vi "Alarm Clock.vi"() -> ()   [LabVIEW 2015]
uses:
  Control 1.ctl
panel:
  in  "Alarm Time":timestamp
  out "Alarm set for":timestamp
  out "Current Time":timestamp
  in  "Turn OFF":bool
  in  "OFF":bool
  in  "Set Alarm":bool
  in  "Snooze":bool
  out "Alarm":bool
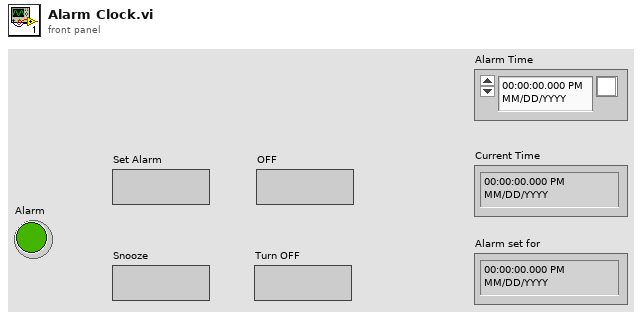
[diagram p1: front panel]
types:
  T1 = typedef "Control 1.ctl" = enum16{"Evaluate", "Set Alarm", "Alarm on", "Alarm off", "Snooze"}
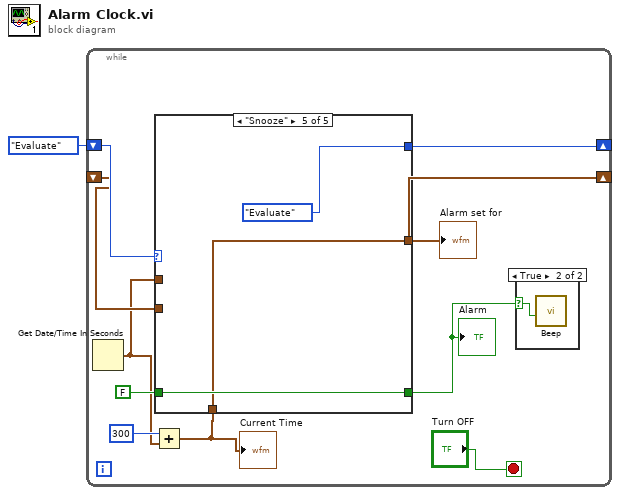
[diagram p0: block diagram]
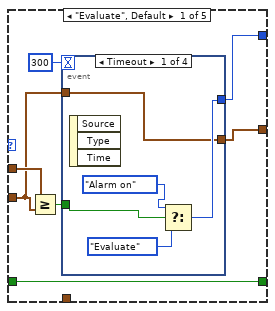
[diagram p3: hidden frame]
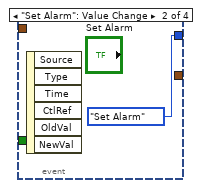
[diagram p4: hidden frame]
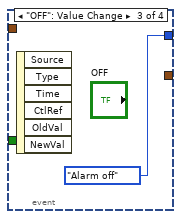
[diagram p5: hidden frame]
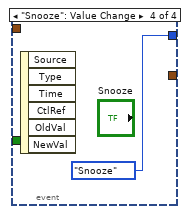
[diagram p6: hidden frame]
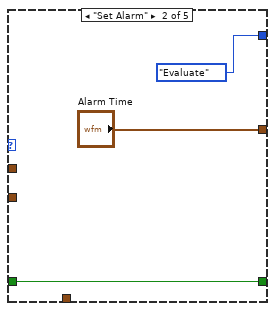
[diagram p7: hidden frame]
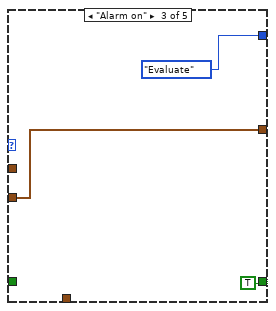
[diagram p8: hidden frame]
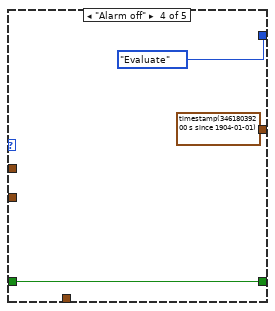
[diagram p9: hidden frame]
diagram:
  n1 = while {
    shift-right: [w9] -> _
    shift-left: Control_1."Evaluate" -> [w11]
    shift-right: [w10] -> _
    shift-left: _ -> [w8]
    stop <- "Turn OFF" stop-if-true
    n2 = Get Date/Time In Seconds() -> (seconds since 1Jan1904=w4:timestamp)
    n3 = Add(x=300, y=w4) -> (x+y=w3:timestamp)
    "Current Time" <- w3
    n4 = case shown="\"Snooze\"" w11 {
      tunnel: [w13 "Alarm Time" w32 timestamp(34618039200 s since 1904-01-01) ("Alarm Time") w37] -> w10
      tunnel: [w18 Control_1."Evaluate" Control_1."Evaluate" Control_1."Evaluate" Control_1."Evaluate"] -> w9
      tunnel: w8 -> [w14 _ w32 _ _]
      tunnel: [w16 w29 TRUE w36 w39] -> w2
      tunnel: FALSE -> [w16 w29 _ w36 w39]
      tunnel: w4 -> [w15 _ _ _ _]
      tunnel: w3 -> [_ _ _ _ w37]
      frame "Evaluate", Default {
        n5 = Greater Or Equal?(x=w15, y=w14) -> (x >= y?=w17:bool)
        n6 = event shown="[0] Timeout" {
          selector: _ -> [_ _ _ _]
          dyn-events: _ -> [_ _ _ _]
          timeout: 300 -> [_ _ _ _]
          tunnel: [w22 Control_1."Set Alarm" Control_1."Alarm off" Control_1."Snooze"] -> w18
          tunnel: w17 -> [w21 _ _ _]
          tunnel: w14 -> [w20 _ _ _]
          tunnel: [w20 _ _ _] -> w13
          event Timeout {
            n7 = event-data() -> ()  [unwired: 1 in, 3 out]
            n8 = Select(t=Control_1."Alarm on", s=w21, f=Control_1."Evaluate") -> (s? t:f=w22:T1)
          }
          event "Set Alarm": Value Change {
            n9 = event-data() -> ()  [unwired: 1 in, 6 out]
          }
          event "OFF": Value Change {
            n10 = event-data() -> ()  [unwired: 1 in, 6 out]
          }
          event "Snooze": Value Change {
            n11 = event-data() -> ()  [unwired: 1 in, 6 out]
          }
        }
      }
      frame "Set Alarm" {
      }
      frame "Alarm on" {
      }
      frame "Alarm off" {
      }
      frame "Snooze" {
      }
    }
    "Alarm set for" <- w10
    "Alarm" <- w2
    n12 = case shown="True" w2 {
      selector: w2 -> [_ w12]
      frame False {
      }
      frame True {
        n13 = call <vilib>:"Beep.vi"("use system alert? (T)"=w12) -> ()  [unwired: 11 in]
      }
    }
  }
